vi "Control AlgorithmV2.vi"(5 "Motor to Control":dbl, 8 "Manual Control":bool, 9 "Angles In":dbl[](array[numeric]), 10 "JoystickIn":i32[](array[numeric])) -> (2 "Target Angles":dbl[](array[numeric]), 3 "MotorsOut":u16[](array[numeric]))   [LabVIEW 2013, in "ProcessorHelperFunctions.lvlib"]
uses:
  ProcessorHelperFunctions.lvlib
panel:
  in  "D gain":dbl
  in  "I Gain":dbl
  in  "Pgain":dbl=1.5
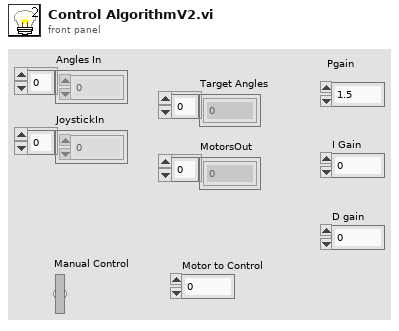
[diagram p1: front panel]
types:
  T1 = cluster{"JoystickIn[0]":i32, "JoystickIn[1]":i32, "JoystickIn[2]":i32, "JoystickIn[3]":i32, "JoystickIn[4]":i32, "JoystickIn[5]":i32, "JoystickIn[6]":i32, "JoystickIn[7]":i32, "JoystickIn[8]":i32, "JoystickIn[9]":i32}
  T2 = cluster{"Angles In[0]":dbl, "Angles In[1]":dbl, "Angles In[2]":dbl, "Angles In[3]":dbl}
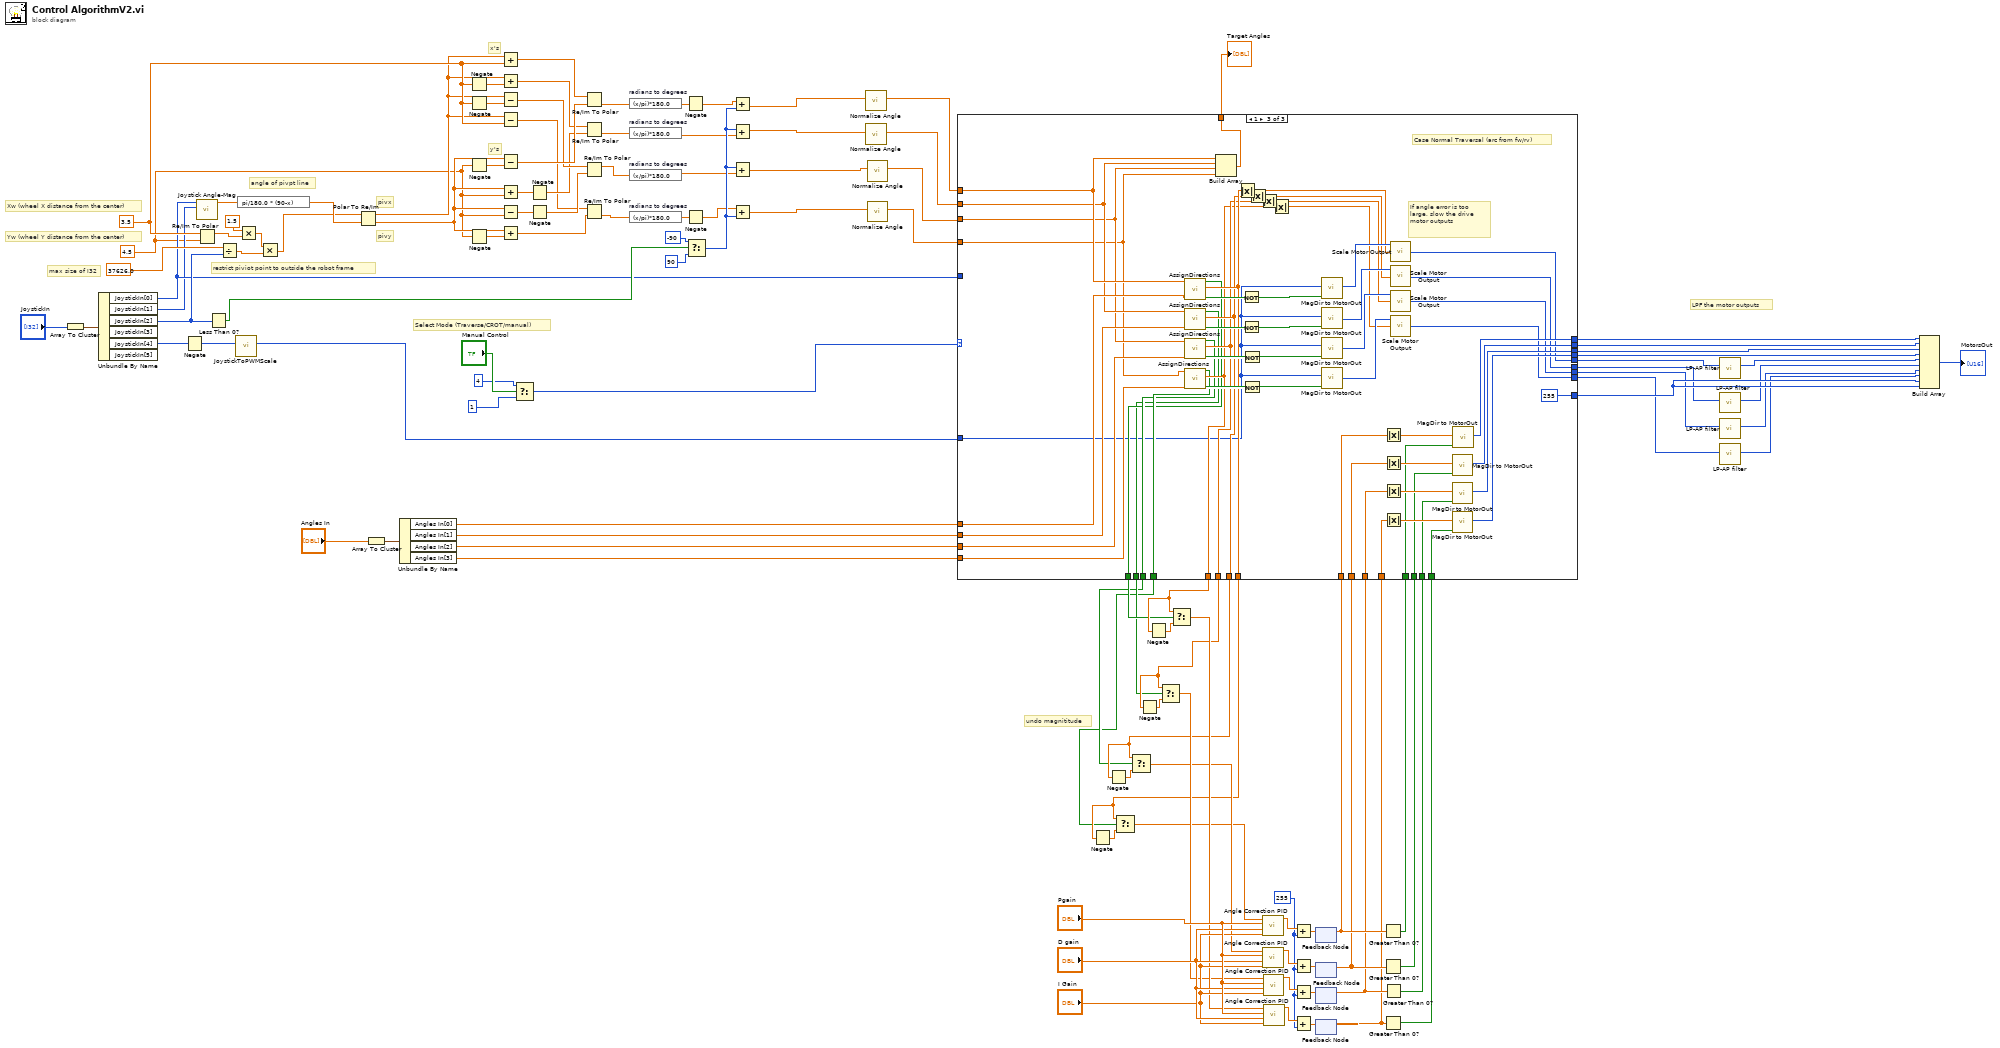
[diagram p0: block diagram]
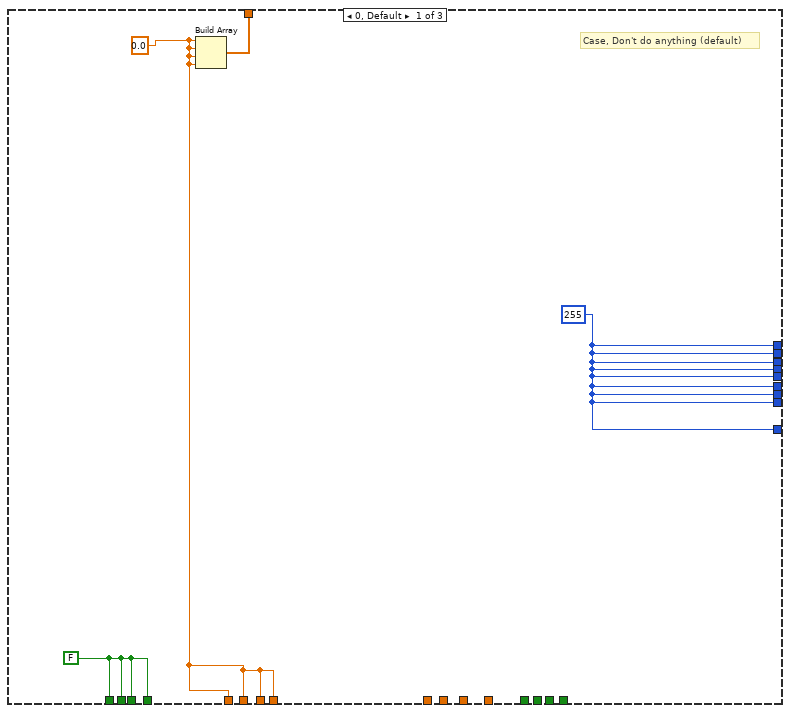
[diagram p2: hidden frame]
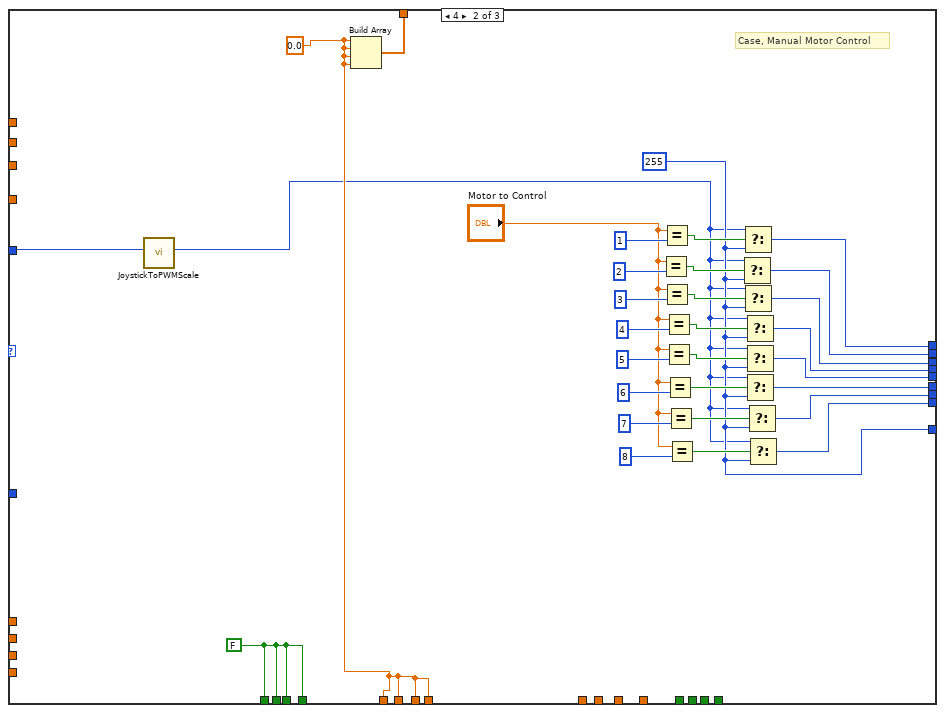
[diagram p3: hidden frame]
diagram:
  w22 = 4.5
  w61 = 3.5
  w9 = 255
  # "max size of I32"
  # "y's"
  # "x's"
  # "restrict piviot point to outside the robot frame"
  # "Yw (wheel Y distance from the center)"
  # "Xw (wheel X distance from the center)"
  # "pivy"
  # "pivx"
  # "angle of pivpt line"
  # "undo magnititude"
  # "LPF the motor outputs"
  # "Select Mode (Traverse/CROT/manual)"
  n1 = Array To Cluster(array="JoystickIn") -> (cluster=w116:T1)
  n2 = Unbundle By Name(w116) -> ("JoystickIn[0]"=w44:i32, "JoystickIn[1]"=w43:i32, "JoystickIn[2]"=w56:i32, "JoystickIn[4]"=w58:i32)  [unwired: 2 out]
  n3 = Negate(x=w58) -> (-x=w51:i32)
  n4 = call "Joystick Angle-Mag.vi"("Yaxis"=w43, "Xaxis"=w44) -> ("Angle"=w66:dbl)  [unwired: 8 in, 1 out]
  n5 = Re/Im To Polar(2:w22, 3:w61) -> (1:w64:dbl)  [unwired: 1 out]
  n6 = Less Than 0?(x=w56) -> (x < 0?=w52:bool)
  n7 = Divide(x=37626.0, y=w56) -> (x/y=w60:dbl)
  n8 = call "JoystickToPWMScale.vi"("Numeric"=w51) -> ("Numeric 2"=w57:u16)  [unwired: 10 in]
  n9 = expression code="pi/180.0 * (90-x)"(w66) -> (w67:dbl)
  n10 = Multiply(x=1.5, y=w64) -> (x*y=w50:dbl)
  n11 = Multiply(x=w50, y=w60) -> (x*y=w65:dbl)
  n12 = Polar To Re/Im(2:w67, 3:w65) -> (0:w41:dbl, 1:w42:dbl)
  n13 = Array To Cluster(array="Angles In") -> (cluster=w109:T2)
  n14 = Unbundle By Name(w109) -> ("Angles In[0]"=w107:dbl, "Angles In[1]"=w106:dbl, "Angles In[2]"=w105:dbl, "Angles In[3]"=w104:dbl)
  n15 = Negate(x=w61) -> (-x=w21:dbl)
  n16 = Negate(x=w61) -> (-x=w20:dbl)
  n17 = Negate(x=w22) -> (-x=w19:dbl)
  n18 = Negate(x=w22) -> (-x=w18:dbl)
  n19 = Add(x=w42, y=w61) -> (x+y=w16:dbl)
  n20 = Add(x=w42, y=w21) -> (x+y=w28:dbl)
  n21 = Subtract(x=w42, y=w20) -> (x-y=w27:dbl)
  n22 = Subtract(x=w42, y=w61) -> (x-y=w17:dbl)
  n23 = Subtract(x=w41, y=w19) -> (x-y=w63:dbl)
  n24 = Add(x=w41, y=w22) -> (x+y=w26:dbl)
  n25 = Subtract(x=w41, y=w22) -> (x-y=w25:dbl)
  n26 = Add(x=w41, y=w18) -> (x+y=w62:dbl)
  n27 = Select(t=4, s="Manual Control", f=1) -> (s? t:f=w102:i32)
  n28 = Negate(x=w26) -> (-x=w24:dbl)
  n29 = Negate(x=w25) -> (-x=w23:dbl)
  n30 = Re/Im To Polar(2:w63, 3:w16) -> (0:w48:dbl)  [unwired: 1 out]
  n31 = Re/Im To Polar(2:w24, 3:w28) -> (0:w47:dbl)  [unwired: 1 out]
  n32 = Re/Im To Polar(2:w23, 3:w27) -> (0:w46:dbl)  [unwired: 1 out]
  n33 = Re/Im To Polar(2:w62, 3:w17) -> (0:w45:dbl)  [unwired: 1 out]
  n34 = expression code="(x/pi)*180.0" "radians to degrees"(w48) -> (w32:dbl)
  n35 = expression code="(x/pi)*180.0" "radians to degrees"(w47) -> (w31:dbl)
  n36 = expression code="(x/pi)*180.0" "radians to degrees"(w46) -> (w30:dbl)
  n37 = expression code="(x/pi)*180.0" "radians to degrees"(w45) -> (w29:dbl)
  n38 = Negate(x=w32) -> (-x=w15:dbl)
  n39 = Negate(x=w29) -> (-x=w14:dbl)
  n40 = Select(t=-90, s=w52, f=90) -> (s? t:f=w55:i32)
  n41 = Add(x=w15, y=w55) -> (x+y=w40:dbl)
  n42 = Add(x=w55, y=w31) -> (x+y=w37:dbl)
  n43 = Add(x=w55, y=w30) -> (x+y=w38:dbl)
  n44 = Add(x=w14, y=w55) -> (x+y=w39:dbl)
  n45 = call "Normalize Angle.vi"("Input"=w40) -> ("Output"=w36:dbl)  [unwired: 10 in]
  n46 = call "Normalize Angle.vi"("Input"=w37) -> ("Output"=w35:dbl)  [unwired: 10 in]
  n47 = call "Normalize Angle.vi"("Input"=w38) -> ("Output"=w34:dbl)  [unwired: 10 in]
  n48 = call "Normalize Angle.vi"("Input"=w39) -> ("Output"=w33:dbl)  [unwired: 10 in]
  n49 = feedback #1() -> (w8:dbl)  [unwired: 1 in]
  n50 = feedback #2() -> (w7:dbl)  [unwired: 1 in]
  n51 = feedback #3() -> (w6:dbl)  [unwired: 1 in]
  n52 = feedback #4() -> (w5:dbl)  [unwired: 1 in]
  n53 = Greater Than 0?(x=w8) -> (x > 0?=w4:bool)
  n54 = Greater Than 0?(x=w7) -> (x > 0?=w3:bool)
  n55 = Greater Than 0?(x=w5) -> (x > 0?=w1:bool)
  n56 = Greater Than 0?(x=w6) -> (x > 0?=w2:bool)
  n57 = case shown="1" w102 {
    tunnel: [w121 w149 w203] -> w114
    tunnel: [w121 w134 w202] -> w113
    tunnel: [w121 w133 w201] -> w112
    tunnel: [w121 w132 w200] -> w111
    tunnel: [w121 w127 255] -> w110
    tunnel: [w121 w131 w170] -> w99
    tunnel: [w121 w130 w169] -> w97
    tunnel: [w121 w129 w168] -> w95
    tunnel: [w121 w128 w167] -> w93
    tunnel: w107 -> [_ _ w190]
    tunnel: w106 -> [_ _ w189]
    tunnel: w105 -> [_ _ w188]
    tunnel: w104 -> [_ _ w187]
    tunnel: w44 -> [_ w123 _]
    tunnel: [w120 w152 w186] -> w103
    tunnel: [w119 w125 w185] -> w69
    tunnel: [w119 w125 w184] -> w73
    tunnel: [w119 w125 w183] -> w76
    tunnel: [w119 w125 w182] -> w79
    tunnel: w8 -> [_ _ w181]
    tunnel: w7 -> [_ _ w180]
    tunnel: w6 -> [_ _ w179]
    tunnel: w5 -> [_ _ w178]
    tunnel: [w118 w124 w177] -> w10
    tunnel: [w118 w124 w176] -> w11
    tunnel: [w118 w124 w174] -> w12
    tunnel: [w118 w124 w175] -> w13
    tunnel: w57 -> [_ _ w165]
    tunnel: w36 -> [_ _ w164]
    tunnel: w35 -> [_ _ w163]
    tunnel: w34 -> [_ _ w162]
    tunnel: w33 -> [_ _ w161]
    tunnel: w4 -> [_ _ w156]
    tunnel: w3 -> [_ _ w155]
    tunnel: w2 -> [_ _ w154]
    tunnel: w1 -> [_ _ w153]
    frame 0, Default {
      w118 = FALSE
      w119 = 0.0
      w121 = 255
      # "Case, Don't do anything (default)"
      n58 = Build Array(w119, w119, w119, w119) -> (w120:dbl[])
    }
    frame 4 {
      w124 = FALSE
      w127 = 255
      w125 = 0.0
      # "Case, Manual Motor Control"
      n59 = call "JoystickToPWMScale.vi"("Numeric"=w123) -> ("Numeric 2"=w122:u16)  [unwired: 10 in]
      n60 = Build Array(w125, w125, w125, w125) -> (w152:dbl[])
      n61 = Equal?(x="Motor to Control", y=2) -> (x = y?=w147:bool)
      n62 = Equal?(x="Motor to Control", y=1) -> (x = y?=w150:bool)
      n63 = Equal?(x="Motor to Control", y=3) -> (x = y?=w145:bool)
      n64 = Equal?(x="Motor to Control", y=4) -> (x = y?=w143:bool)
      n65 = Equal?(x="Motor to Control", y=5) -> (x = y?=w141:bool)
      n66 = Equal?(x="Motor to Control", y=6) -> (x = y?=w139:bool)
      n67 = Equal?(x="Motor to Control", y=7) -> (x = y?=w137:bool)
      n68 = Equal?(x="Motor to Control", y=8) -> (x = y?=w135:bool)
      n69 = Select(t=w122, s=w147, f=w127) -> (s? t:f=w134:i32)
      n70 = Select(t=w122, s=w150, f=w127) -> (s? t:f=w149:i32)
      n71 = Select(t=w122, s=w145, f=w127) -> (s? t:f=w133:i32)
      n72 = Select(t=w122, s=w143, f=w127) -> (s? t:f=w132:i32)
      n73 = Select(t=w122, s=w141, f=w127) -> (s? t:f=w131:i32)
      n74 = Select(t=w122, s=w139, f=w127) -> (s? t:f=w130:i32)
      n75 = Select(t=w122, s=w137, f=w127) -> (s? t:f=w129:i32)
      n76 = Select(t=w122, s=w135, f=w127) -> (s? t:f=w128:i32)
    }
    frame 1 {
      # "Case Normal Traversal (arc from fw/rv)"
      # "If angle error is too large, slow the drive motor outputs"
      n77 = call "AssignDirections.vi"("Actual Angle"=w190, "Target Angle"=w164) -> ("Reverse Wheel Direction"=w207:bool, "Lowest Angle Error"=w185:dbl, "Turn Clockwise"=w175:bool)  [unwired: 7 in]
      n78 = call "AssignDirections.vi"("Actual Angle"=w189, "Target Angle"=w163) -> ("Reverse Wheel Direction"=w206:bool, "Lowest Angle Error"=w184:dbl, "Turn Clockwise"=w174:bool)  [unwired: 7 in]
      n79 = call "AssignDirections.vi"("Actual Angle"=w188, "Target Angle"=w162) -> ("Reverse Wheel Direction"=w205:bool, "Lowest Angle Error"=w183:dbl, "Turn Clockwise"=w176:bool)  [unwired: 7 in]
      n80 = call "AssignDirections.vi"("Actual Angle"=w187, "Target Angle"=w161) -> ("Reverse Wheel Direction"=w204:bool, "Lowest Angle Error"=w182:dbl, "Turn Clockwise"=w177:bool)  [unwired: 7 in]
      n81 = Build Array(w164, w163, w162, w161) -> (w186:dbl[])
      n82 = Absolute Value(x=w185) -> (abs(x)=w173:dbl)
      n83 = Not(x=w207) -> (.not. x?=w191:bool)
      n84 = Not(x=w206) -> (.not. x?=w192:bool)
      n85 = Not(x=w205) -> (.not. x?=w193:bool)
      n86 = Not(x=w204) -> (.not. x?=w194:bool)
      n87 = Absolute Value(x=w184) -> (abs(x)=w166:dbl)
      n88 = Absolute Value(x=w183) -> (abs(x)=w172:dbl)
      n89 = Absolute Value(x=w182) -> (abs(x)=w171:dbl)
      n90 = call "MagDir to MotorOut.vi"("Fwd. Dir?"=w191, "Input"=w165) -> ("Output"=w198:i16)  [unwired: 9 in]
      n91 = call "MagDir to MotorOut.vi"("Fwd. Dir?"=w192, "Input"=w165) -> ("Output"=w197:i16)  [unwired: 9 in]
      n92 = call "MagDir to MotorOut.vi"("Fwd. Dir?"=w193, "Input"=w165) -> ("Output"=w196:i16)  [unwired: 9 in]
      n93 = call "MagDir to MotorOut.vi"("Fwd. Dir?"=w194, "Input"=w165) -> ("Output"=w195:i16)  [unwired: 9 in]
      n94 = Absolute Value(x=w181) -> (abs(x)=w160:dbl)
      n95 = Absolute Value(x=w180) -> (abs(x)=w159:dbl)
      n96 = Absolute Value(x=w179) -> (abs(x)=w158:dbl)
      n97 = Absolute Value(x=w178) -> (abs(x)=w157:dbl)
      n98 = call "Scale Motor Output.vi"("Error Input"=w173, "Motor Input"=w198) -> ("Output"=w170:u32)  [unwired: 1 in]
      n99 = call "Scale Motor Output.vi"("Error Input"=w166, "Motor Input"=w197) -> ("Output"=w169:u32)  [unwired: 1 in]
      n100 = call "Scale Motor Output.vi"("Error Input"=w172, "Motor Input"=w196) -> ("Output"=w168:u32)  [unwired: 1 in]
      n101 = call "Scale Motor Output.vi"("Error Input"=w171, "Motor Input"=w195) -> ("Output"=w167:u32)  [unwired: 1 in]
      n102 = call "MagDir to MotorOut.vi"("Fwd. Dir?"=w155, "Input"=w159) -> ("Output"=w202:i16)  [unwired: 9 in]
      n103 = call "MagDir to MotorOut.vi"("Fwd. Dir?"=w154, "Input"=w158) -> ("Output"=w201:i16)  [unwired: 9 in]
      n104 = call "MagDir to MotorOut.vi"("Fwd. Dir?"=w153, "Input"=w157) -> ("Output"=w200:i16)  [unwired: 9 in]
      n105 = call "MagDir to MotorOut.vi"("Fwd. Dir?"=w156, "Input"=w160) -> ("Output"=w203:i16)  [unwired: 9 in]
    }
  }
  "Target Angles" <- w103
  n106 = Negate(x=w69) -> (-x=w71:dbl)
  n107 = Negate(x=w73) -> (-x=w74:dbl)
  n108 = Select(t=w69, s=w10, f=w71) -> (s? t:f=w70:dbl)
  n109 = Select(t=w73, s=w11, f=w74) -> (s? t:f=w72:dbl)
  n110 = Negate(x=w76) -> (-x=w77:dbl)
  n111 = Negate(x=w79) -> (-x=w80:dbl)
  n112 = Select(t=w76, s=w12, f=w77) -> (s? t:f=w75:dbl)
  n113 = Select(t=w79, s=w13, f=w80) -> (s? t:f=w78:dbl)
  n114 = call "Angle Correction PID.vi"("I gain"="I Gain", "D gain"="D gain", "P gain"="Pgain", "Error In"=w70) -> ("Output"=w87:dbl)  [unwired: 7 in]
  n115 = call "Angle Correction PID.vi"("I gain"="I Gain", "D gain"="D gain", "P gain"="Pgain", "Error In"=w72) -> ("Output"=w86:dbl)  [unwired: 7 in]
  n116 = call "Angle Correction PID.vi"("I gain"="I Gain", "D gain"="D gain", "P gain"="Pgain", "Error In"=w75) -> ("Output"=w85:dbl)  [unwired: 7 in]
  n117 = call "Angle Correction PID.vi"("I gain"="I Gain", "D gain"="D gain", "P gain"="Pgain", "Error In"=w78) -> ("Output"=w84:dbl)  [unwired: 7 in]
  n118 = Add(x=w87, y=w9) -> (x+y=w91:dbl)
  n119 = Add(x=w86, y=w9) -> (x+y=w90:dbl)
  n120 = Add(x=w85, y=w9) -> (x+y=w89:dbl)
  n121 = Add(x=w84, y=w9) -> (x+y=w88:dbl)
  n122 = feedback-in #1(w91) -> ()
  n123 = feedback-in #2(w90) -> ()
  n124 = feedback-in #3(w89) -> ()
  n125 = feedback-in #4(w88) -> ()
  n126 = call "LP-AP filter.vi"("Input"=w99) -> ("Output"=w98:u16)  [unwired: 9 in, 1 out]
  n127 = call "LP-AP filter.vi"("Input"=w97) -> ("Output"=w96:u16)  [unwired: 9 in, 1 out]
  n128 = call "LP-AP filter.vi"("Input"=w95) -> ("Output"=w94:u16)  [unwired: 9 in, 1 out]
  n129 = call "LP-AP filter.vi"("Input"=w93) -> ("Output"=w92:u16)  [unwired: 9 in, 1 out]
  n130 = Build Array(w114, w113, w112, w111, w98, w96, w94, w92, w110, w110) -> (→"MotorsOut":i32[])
